vi "Exmples.vi"(8 "error in (no error)":errorcluster) -> (0 "error out":errorcluster)   [LabVIEW 2021, in "Markdown.lvlib"]
doc: "Exports the example VIs (i.e. Starts with \"Example*.vi\") block diagram images."
uses:
  Markdown.lvlib
  Global.vi
  <vilib>/Utility/error.llb/Error Cluster From Error Code.vi
  <vilib>/ErrorRing/Error Ring.xnode
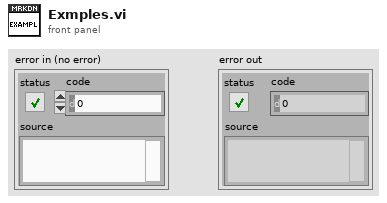
[diagram p1: front panel]
types:
  T1 = typedef "Markdown.lvlib/Item.ctl" = cluster{"Name":string, "Icon":picture, "Path":path, "Title":string, "Desc":string, "ConPane":picture, "TypeString":string, "ProjectItem":string, "VI Type":enum32{"invalid VI type", "Standard VI", "Control VI", "Global VI", "Polymorphic VI", "Configuration VI", "SubSystem", "Facade VI", "Method VI", "Statechart Diagram VI"}}
  T2 = typedef "imagedata.ctl" = cluster{"image type":i32, "image depth":i32, "image":u8[], "mask":u8[], "colors":u32[], "Rectangle":cluster{"left":i16, "top":i16, "right":i16, "bottom":i16}}
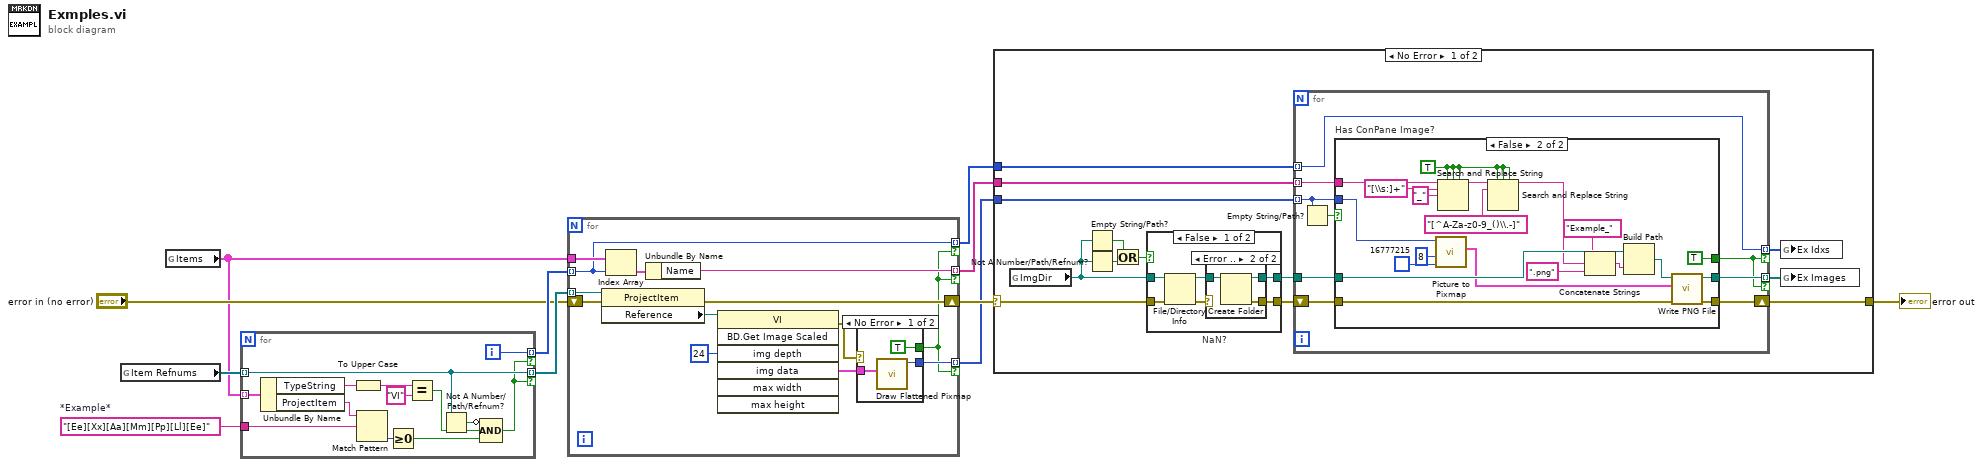
[diagram p0: block diagram]
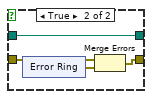
[diagram p4: hidden frame]
diagram:
  w4 = "[Ee][Xx][Aa][Mm][Pp][Ll][Ee]"  # *Example*
  n1 = global read "Global.vi" "Item Refnums"() -> (w2:refnum<vi>[])
  n2 = global read "Global.vi" "Items"() -> (w1:T1[])
  n3 = for {
    tunnel: w1 -> [w24] mode=indexing
    tunnel: w4 -> [w22]
    tunnel: [w14] -> w10 mode=indexing if=w12
    tunnel: w2 -> [w14] mode=indexing
    tunnel: [w13] -> w11 mode=indexing if=w12
    i -> [w13]
    n4 = Unbundle By Name(w24) -> ("TypeString"=w19:string, "ProjectItem"=w21:string)
    n5 = To Upper Case(1:w19) -> (0:w18:string)
    n6 = Match Pattern(string=w21, regular expression=w22) -> (offset past match=w23:i32)  [unwired: 1 in, 3 out]
    n7 = Greater Or Equal To 0?(x=w23) -> (x >= 0?=w20:bool)
    n8 = Equal?(x=w18, y="VI") -> (x = y?=w16:bool)
    n9 = Not A Number/Path/Refnum?(number/path/refnum=w14) -> (NaN/Path/Refnum?=w15:bool)
    n10 = Compound Arithmetic op=AND(invert w15, w16, w20) -> (w12:bool)
  }
  n11 = for {
    tunnel: w1 -> [w31]
    shift-right: [w28] -> w9
    shift-left: "error in (no error)" -> [w37]
    tunnel: [w29] -> w6 mode=indexing if=w25
    tunnel: [w32] -> w7 mode=indexing if=w25
    tunnel: w11 -> [w26] mode=indexing
    tunnel: w10 -> [w35] mode=indexing
    tunnel: [w26] -> w3 mode=indexing if=w25
    n12 = property class="ProjectItem"(reference=w35, error in=w37) -> (error out=w28:errorcluster, "Reference"=w36:refnum<vi>)  [unwired: 1 out]
    n13 = Index Array(array=w31, index=w26) -> (element=w30:T1)
    n14 = Unbundle By Name(w30) -> ("Name"=w29:string)
    n15 = invoke class="VI" method="BD.Get Image Scaled"(reference=w36, "img depth"=24 ("Image Depth")) -> (error out=w27:errorcluster, "img data"=w33:T2)  [unwired: 5 in, 5 out]
    n16 = case shown="No Error" w27 {
      tunnel: w33 -> [w40 _]
      tunnel: [w39 _] -> w32
      tunnel: [TRUE _] -> w25
      frame No Error {
        n17 = call <vilib>:"Draw Flattened Pixmap.vi"("image data"=w40) -> ("new picture"=w39:picture)  [unwired: 8 in]
      }
      frame Error {
      }
    }
  }
  n18 = case shown="No Error" w9 {
    selector: w9 -> [w53 w103]
    tunnel: [w52 w103] -> w5
    tunnel: w7 -> [w46 _]
    tunnel: w6 -> [w45 _]
    tunnel: w3 -> [w44 _]
    frame No Error {
      n19 = global read "Global.vi" "ImgDir"() -> (w43:path)
      n20 = Empty String/Path?(string/path=w43) -> (empty?=w48:bool)
      n21 = Not A Number/Path/Refnum?(number/path/refnum=w43) -> (NaN/Path/Refnum?=w49:bool)
      n22 = Or(x=w48, y=w49) -> (x .or. y?=w47:bool)
      n23 = case "NaN?" shown="False" w47 {
        tunnel: w53 -> [w59 w68]
        tunnel: w43 -> [w57 w67]
        tunnel: [w56 w66] -> w51
        tunnel: [w54 w67] -> w50
        frame False {
          n24 = File/Directory Info(path=w57, error in=w59) -> (path out=w55:path, error out=w58:errorcluster)  [unwired: 5 out]
          n25 = case shown="Error .." w58 {
            selector: w58 -> [w60 _]
            tunnel: [w60 w64] -> w56
            tunnel: w55 -> [w61 w63]
            tunnel: [w61 w62] -> w54
            frame No Error {
            }
            frame Error {
              n26 = Create Folder(path (use dialog)=w63) -> (created path=w62:path, error out=w64:errorcluster)  [unwired: 2 in, 1 out]
            }
          }
        }
        frame True {
          n27 = xnode "Error Ring"() -> ("error out"=w65:errorcluster)
          n28 = Merge Errors(w68, w65) -> (w66:errorcluster)
        }
      }
      n29 = for {
        shift-right: [w81] -> w52
        shift-left: w51 -> [w77]
        tunnel: [w80] -> w41 mode=indexing if=w76
        tunnel: w50 -> [w79]
        tunnel: [w73] -> w42 mode=indexing if=w76
        tunnel: w46 -> [w75] mode=indexing
        tunnel: w45 -> [w74] mode=indexing
        tunnel: w44 -> [w73] mode=indexing
        n30 = Empty String/Path?(string/path=w75) -> (empty?=w78:bool)
        n31 = case "Has ConPane Image?" shown="False" w78 {
          tunnel: w77 -> [w82 w98]
          tunnel: [w82 w102] -> w81
          tunnel: [_ w100] -> w80
          tunnel: w79 -> [_ w99]
          tunnel: w74 -> [_ w85]
          tunnel: w75 -> [_ w87]
          tunnel: [_ TRUE] -> w76
          frame True {
          }
          frame False {
            w88 = TRUE ("replace all? (F)")
            n32 = call <vilib>:"Picture to Pixmap.vi"("Background Color"=u32 16777215, "depth"=8, "picture"=w87) -> ("image data"=w86:T2)  [unwired: 7 in, 1 out]
            n33 = Search and Replace String(replace all?=w88, case sensitive?=w88, multiline?=w88, input string=w85, search string="[\\s:]+", replace string="_" ("replace string (\"\")")) -> (result string=w91:string)  [unwired: 2 in, 3 out]
            n34 = Search and Replace String(replace all?=w88, case sensitive?=w88, multiline?=w88, input string=w91, search string="[^A-Za-z0-9_()\\.-]") -> (result string=w92:string)  [unwired: 3 in, 3 out]
            n35 = Concatenate Strings("Example_" ("string"), w92, ".png" ("string")) -> (w84:string)
            n36 = Build Path(base path=w99, name or relative path=w84) -> (appended path=w101:path)
            n37 = call <vilib>:"Write PNG File.vi"("error in (no error)"=w98, "image data"=w86, "path to PNG file"=w101) -> ("error out"=w102:errorcluster, "path"=w100:path)  [unwired: 7 in]
          }
        }
      }
      n38 = global write "Global.vi" "Ex Idxs"(w42) -> ()
      n39 = global write "Global.vi" "Ex Images"(w41) -> ()
    }
    frame Error {
    }
  }
  "error out" <- w5
